vi "R30.vi"() -> ()   [LabVIEW 2016, in "Beamline Sections.lvlib"]
uses:
  Beamline Sections.lvlib
panel:
  out "error out":errorcluster
  in  "Tab Control":enum32{"Controls", "Readbacks"}(tab)
  in  "Y Steerer magnetic":dbl(knob) min=-3.0 max=3.0
  in  "stop":bool
  out "R30 steer Y mag read":dbl=-0.4902823381440002 format="%#_3g"
  out "Y steerer":bool=TRUE
  out "ESA":bool=TRUE
  out "Esa Read":dbl=0.6593698178774999 min=0.0 max=200.0
  in  "Esa":dbl(knob) min=0.0 max=60.0 scale=45.0..48.0
  in  "R30 Y steerer":dbl(knob) min=-10.0 max=10.0 scale=-5.0..7.0
  in  "R30 Quad A":dbl(knob) min=0.0 max=2.0 scale=0.2..0.7
  in  "R30 X steerer":dbl(knob) min=-10.0 max=10.0 scale=-10.0..10.0
  in  "R30 Quad B":dbl(knob) min=0.0 max=2.0 scale=0.2..0.75
  out "R30 Quad A read":dbl=0.35951642376000004 min=0.0 max=200.0 format="%#_3g"
  out "R30 Quad B read":dbl=0.004890288120000014 min=0.0 max=200.0 format="%#_3g"
  out "R30 quad Range":bool=TRUE
  out "R30 Steerer X Read":dbl=3.8467084990949996 format="%#_5g"
  out "R30 Steerer Y Read":dbl=-1.853906631318 format="%#_4g"
  out "R30 Steerer range\n Steerer range":bool=TRUE
  in  "Cluster":T1
  out "Detector cup":bool
  out "R30 steer -Y Set":dbl=6.976792370644522
  out "R30 steer +Y Set":dbl=3.023207629355478
  out "R30 steer -X Set":dbl=2.889401062392519
  out "R30 steer +X Set":dbl=7.110598937607481
  out "R30 steer -Y":dbl=3.27987955401
  out "R30 steer +Y":dbl=1.425972922692
  out "R30 steer -X":dbl=2.8585968391709997
  out "R30 steer +X":dbl=6.705305338265999
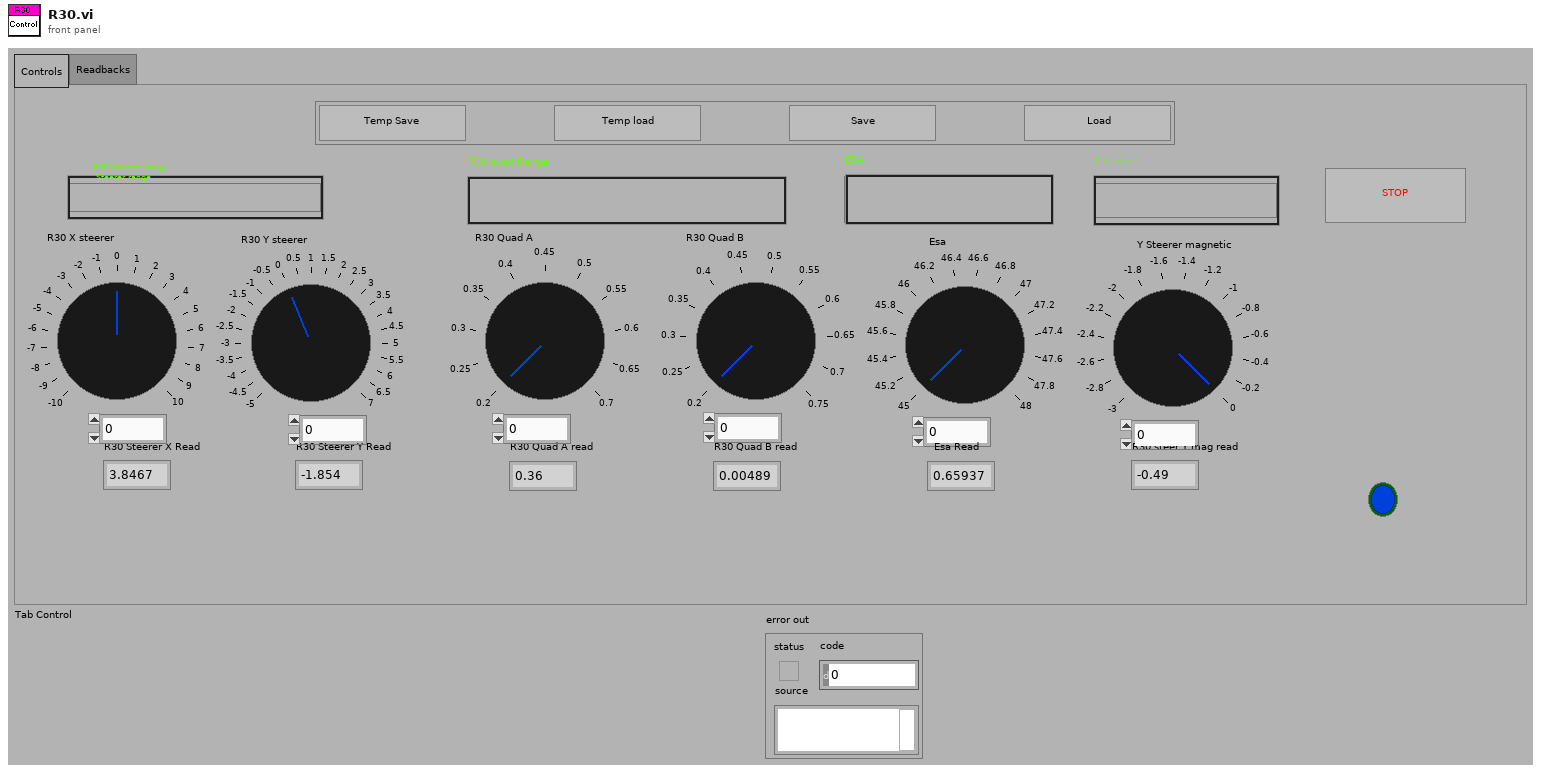
[diagram p1: front panel]
types:
  T1 = cluster{"OK Button":bool, "OK Button 2":bool, "OK Button 3":bool, "OK Button 4":bool}
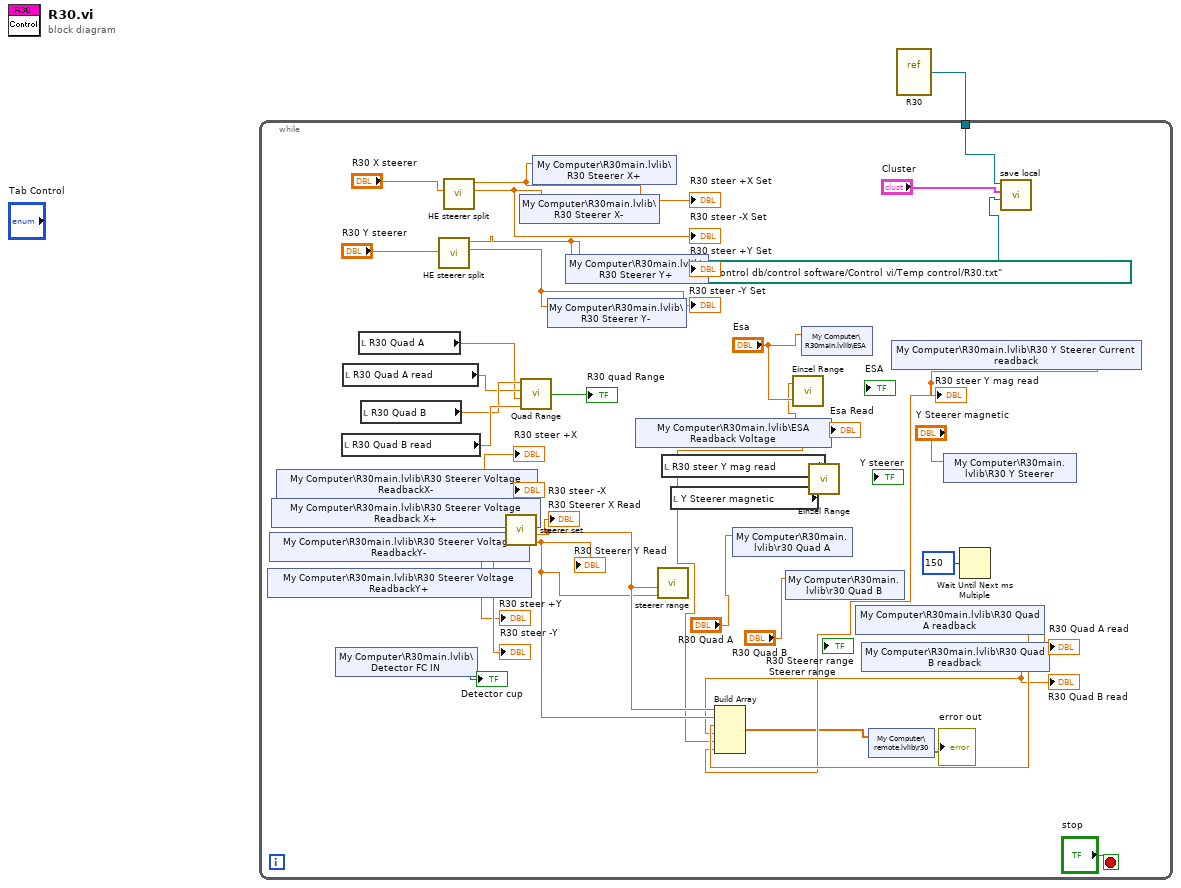
[diagram p0: block diagram]
diagram:
  n1 = vi-ref "R30.vi"() -> (w1:refnum<vi>)
  n2 = while {
    tunnel: w1 -> [w23]
    stop <- "stop" stop-if-true
    n3 = shared-variable "My Computer\\R30main.lvlib\\R30 Steerer Voltage ReadbackY+"() -> (w2:dbl)  [unwired: 1 in, 1 out]
    "R30 steer +Y" <- w2
    n4 = shared-variable "My Computer\\R30main.lvlib\\R30 Steerer Voltage ReadbackY-"() -> (w3:dbl)  [unwired: 1 in, 1 out]
    "R30 steer -Y" <- w3
    n5 = shared-variable "My Computer\\R30main.lvlib\\R30 Steerer Voltage Readback X+"() -> (w17:dbl)  [unwired: 1 in, 1 out]
    "R30 steer +X" <- w17
    n6 = shared-variable "My Computer\\R30main.lvlib\\R30 Steerer Voltage ReadbackX-"() -> (w18:dbl)  [unwired: 1 in, 1 out]
    "R30 steer -X" <- w18
    n7 = shared-variable "My Computer\\R30main.lvlib\\Detector FC IN"() -> (→"Detector cup":bool)  [unwired: 1 in, 1 out]
    n8 = local read "R30 Quad B read"() -> (w35:dbl)
    n9 = local read "R30 Quad A read"() -> (w33:dbl)
    n10 = local read "R30 Quad A"() -> (w32:dbl)
    n11 = local read "R30 Quad B"() -> (w34:dbl)
    n12 = call "HE steerer split.vi"("Steerer in"="R30 Y steerer") -> ("Steerer +"=w20:dbl, "Steerer -"=w19:dbl)  [unwired: 7 out]
    "R30 steer +Y Set" <- w20
    "R30 steer -Y Set" <- w19
    n13 = call "HE steerer split.vi"("Steerer in"="R30 X steerer") -> ("Steerer +"=w22:dbl, "Steerer -"=w21:dbl)  [unwired: 7 out]
    "R30 steer +X Set" <- w22
    "R30 steer -X Set" <- w21
    n14 = call "steerer set.vi"("Injector image X  -"=w18, "Injector image X +"=w17, "Injector image Y  -"=w2, "Injector image Y +"=w3) -> ("Steerer X"=w11:dbl, "Steerer Y"=w10:dbl)  [unwired: 4 out]
    "R30 Steerer X Read" <- w11
    "R30 Steerer Y Read" <- w10
    n15 = shared-variable "My Computer\\R30main.lvlib\\R30 Steerer X-"(w21) -> ()  [unwired: 1 in, 1 out]
    n16 = call "Quad Range.vi"("Transmission Quad B read"=w35, "Transmission Quad A set"=w32, "Transmission Quad A read"=w33, "Transmission Quad B set"=w34) -> ("Quad range?"=→"R30 quad Range":bool)
    n17 = shared-variable "My Computer\\R30main.lvlib\\R30 Steerer X+"(w22) -> ()  [unwired: 1 in, 1 out]
    n18 = shared-variable "My Computer\\R30main.lvlib\\R30 Steerer Y-"(w19) -> ()  [unwired: 1 in, 1 out]
    n19 = shared-variable "My Computer\\R30main.lvlib\\R30 Steerer Y+"(w20) -> ()  [unwired: 1 in, 1 out]
    n20 = shared-variable "My Computer\\R30main.lvlib\\ESA Readback Voltage"() -> (w7:dbl)  [unwired: 1 in, 1 out]
    "Esa Read" <- w7
    n21 = call "steerer range.vi"("Steerer Y Voltage"=w10, "Steerer X Voltage"=w11) -> ()  [unwired: 2 in, 4 out]
    n22 = local read "R30 steer Y mag read"() -> (w31:dbl)
    n23 = local read "Y Steerer magnetic"() -> (w30:dbl)
    n24 = shared-variable "My Computer\\R30main.lvlib\\r30 Quad A"("R30 Quad A") -> ()  [unwired: 1 in, 1 out]
    n25 = shared-variable "My Computer\\R30main.lvlib\\r30 Quad B"("R30 Quad B") -> ()  [unwired: 1 in, 1 out]
    n26 = call "Einzel Range.vi"("Inj image Readback"="Esa", "Inj image Einzel Set"=w7) -> ()  [unwired: 2 out]
    n27 = shared-variable "My Computer\\R30main.lvlib\\ESA"("Esa") -> ()  [unwired: 1 in, 1 out]
    n28 = call "Einzel Range.vi"("Inj image Readback"=w30, "Inj image Einzel Set"=w31) -> ()  [unwired: 2 out]
    n29 = shared-variable "My Computer\\R30main.lvlib\\R30 Quad A readback"() -> (w9:dbl)  [unwired: 1 in, 1 out]
    "R30 Quad A read" <- w9
    n30 = shared-variable "My Computer\\R30main.lvlib\\R30 Quad B readback"() -> (w8:dbl)  [unwired: 1 in, 1 out]
    "R30 Quad B read" <- w8
    n31 = shared-variable "My Computer\\R30main.lvlib\\R30 Y Steerer Current readback"() -> (w6:dbl)  [unwired: 1 in, 1 out]
    "R30 steer Y mag read" <- w6
    n32 = Build Array(w11, w10, w9, w8, w7, w6) -> (w5:dbl[])
    n33 = shared-variable "My Computer\\remote.lvlib\\r30"(w5) -> (error out=→"error out":errorcluster)  [unwired: 1 in]
    n34 = shared-variable "My Computer\\R30main.lvlib\\R30 Y Steerer"("Y Steerer magnetic") -> ()  [unwired: 1 in, 1 out]
    n35 = Wait Until Next ms Multiple(millisecond multiple=u32 150) -> ()  [unwired: 1 out]
    n36 = call "save local.vi"("file path (use dialog)"=path "F:/control db/control software/Control vi/Temp control/R30.txt", "Ring"="Cluster", "VI Refnum"=w23) -> ()  [unwired: 2 out]
  }
